vi "Check station result.vi"(10 "THIS STATION STATUS":string, 11 "PREVIOUS STYATION STATUS":string) -> (1 "CHECKED IN DATABASE FOUND AND FOUND ALREADY TESTED":bool, 2 "CHECKED IN DATABASE FOUND NG":bool, 3 "CHECKED IN DATABASE FOUND OK":bool)   [LabVIEW 2015]
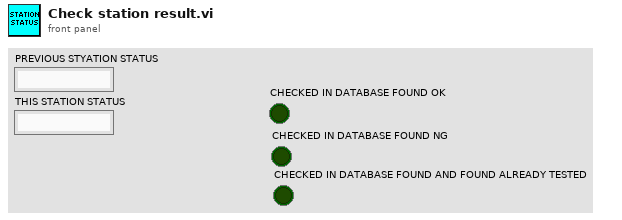
[diagram p1: front panel]
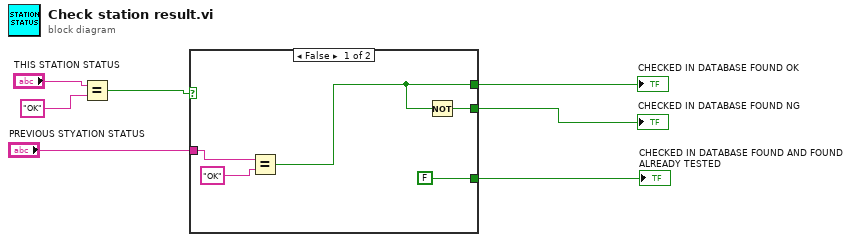
[diagram p0: block diagram]
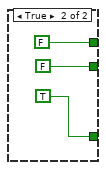
[diagram p2: hidden frame]
diagram:
  n1 = Equal?(x="THIS STATION STATUS", y="OK") -> (x = y?=w5:bool)
  n2 = case shown="False" w5 {
    tunnel: [FALSE TRUE] -> w4
    tunnel: [w8 FALSE] -> w3
    tunnel: [w9 FALSE] -> w2
    tunnel: "PREVIOUS STYATION STATUS" -> [w11 _]
    frame False {
      n3 = Equal?(x=w11, y="OK") -> (x = y?=w9:bool)
      n4 = Not(x=w9) -> (.not. x?=w8:bool)
    }
    frame True {
    }
  }
  "CHECKED IN DATABASE FOUND OK" <- w2
  "CHECKED IN DATABASE FOUND NG" <- w3
  "CHECKED IN DATABASE FOUND AND FOUND ALREADY TESTED" <- w4
